vi "Test Graph.vi"() -> ()   [LabVIEW 2020]
uses:
  <vilib>/Utility/cursorutil.llb/Set Cursor (Icon Pict).vi
  <vilib>/Utility/miscctls.llb/LVPoint32TypeDef.ctl
panel:
  out "x/y":sgl
  in  "数值 2":dbl
  in  "数值":dbl
  in  "最小精度":enum32{"1min", "10s", "1s", "100ms"}(radio)
  in  "Process":bool
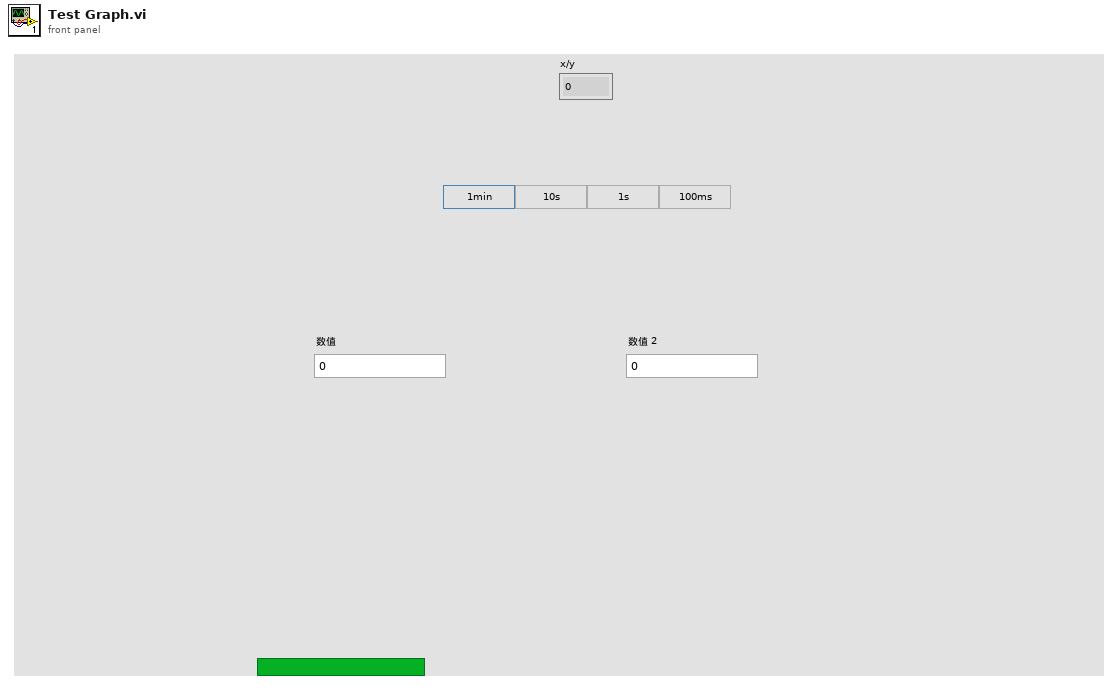
[diagram p1: front panel]
types:
  T1 = typedef "LVPoint32TypeDef.ctl" = cluster{"Horizontal":i32, "Vertical":i32}
  T2 = enum32{"invalid app kind", "Development System", "Run Time System", "Student Edition", "Embedded LabVIEW", "Evaluation", "Custom"}
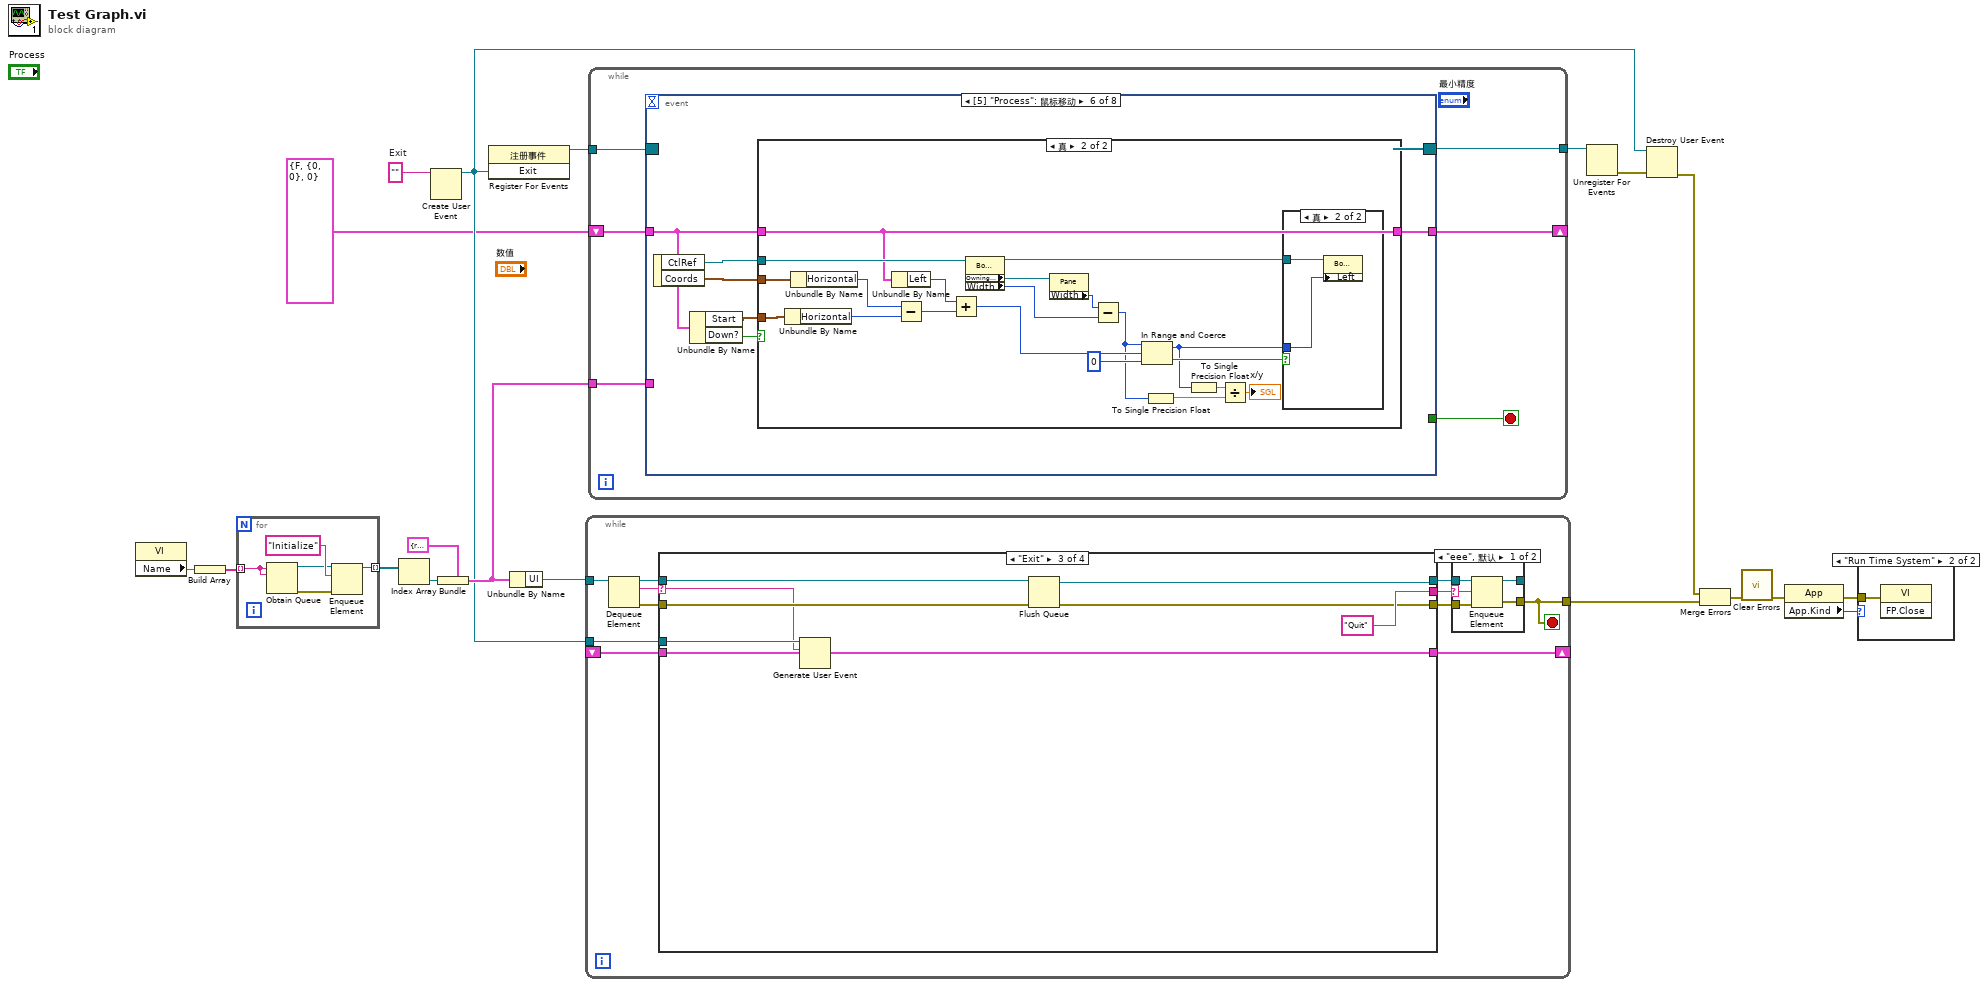
[diagram p0: block diagram]
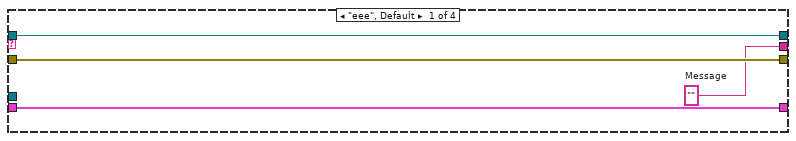
[diagram p4: hidden frame]
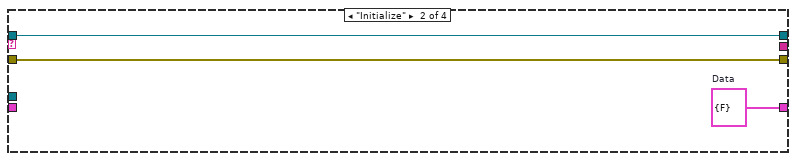
[diagram p5: hidden frame]
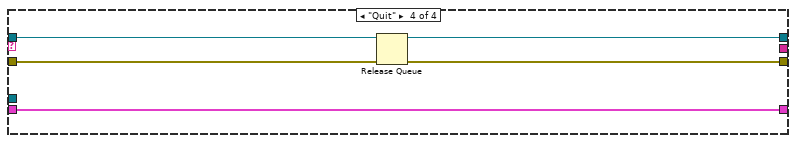
[diagram p6: hidden frame]
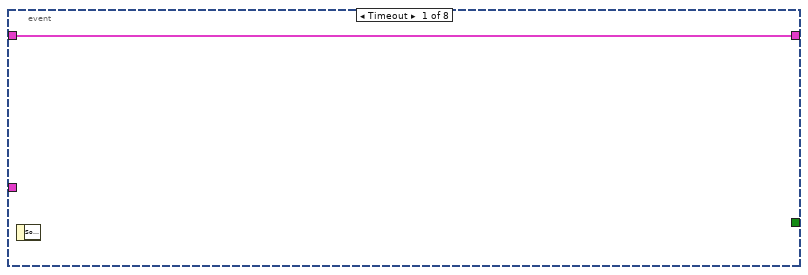
[diagram p7: hidden frame]
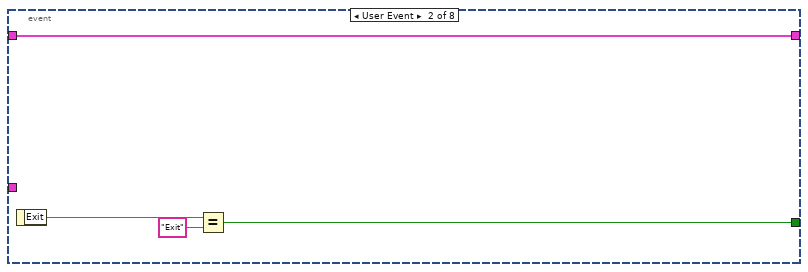
[diagram p8: hidden frame]
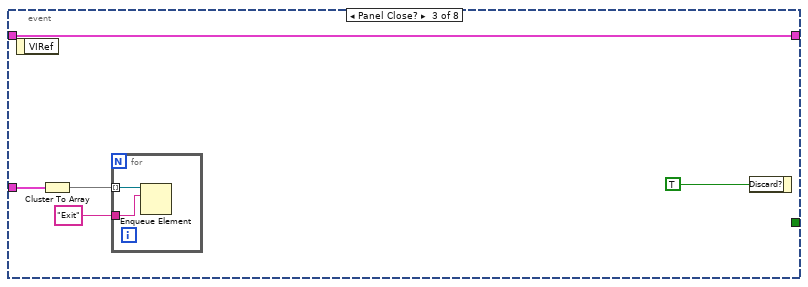
[diagram p9: hidden frame]
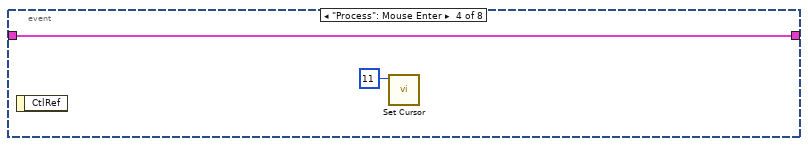
[diagram p10: hidden frame]
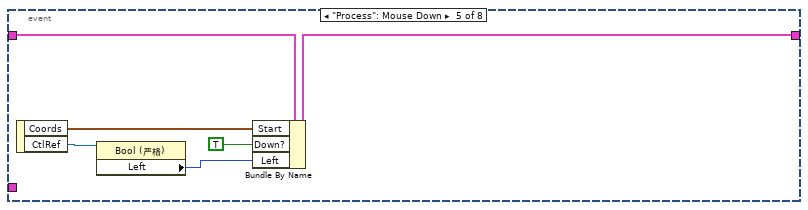
[diagram p11: hidden frame]
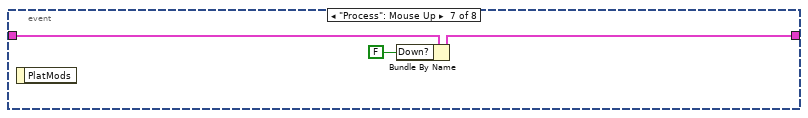
[diagram p14: hidden frame]
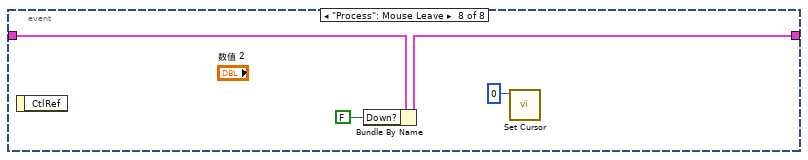
[diagram p15: hidden frame]
diagram:
  w4 = ""  # Exit
  n1 = property class="VI"() -> ("Name"=w14:string)  [unwired: 2 in, 2 out]
  n2 = Build Array(w14) -> (w15:string[])
  n3 = for {
    tunnel: w15 -> [w20] mode=indexing
    tunnel: [w21] -> w9 mode=indexing
    n4 = Obtain Queue(name (unnamed)=w20, element data type=w20) -> (queue out=w23:refnum<queue>, error out=w22:errorcluster)  [unwired: 3 in, 1 out]
    n5 = Enqueue Element(queue=w23, element="Initialize" ("元素"), error in (no error)=w22) -> (queue out=w21:refnum<queue>)  [unwired: 1 in, 2 out]
  }
  n6 = Index Array(array=w9) -> (element=w12:refnum<queue>)  [unwired: 1 in]
  n7 = Create User Event(user event datatype=w4) -> (user event=w8:refnum<user-event>)  [unwired: 1 in, 1 out]
  n8 = Bundle(cluster=cluster{"UI":refnum<queue>} {"UI"=refnum}, "UI"=w12) -> (w13:cluster{"UI":refnum<queue>})
  n9 = register-events(w8) -> (reference out=w5:refnum<event-registration>)  [unwired: 2 in, 1 out]
  n10 = Unbundle By Name(w13) -> ("UI"=w10:refnum<queue>)
  n11 = while {
    tunnel: w10 -> [w35]
    tunnel: [w25] -> w17
    shift-right: [w29] -> _
    shift-left: _ -> [w28]
    tunnel: w8 -> [w27]
    stop <- w25 stop-if-true
    n12 = Dequeue Element(queue=w35) -> (queue out=w34:refnum<queue>, element=w26:string, error out=w31:errorcluster)  [unwired: 2 in, 1 out]
    n13 = case shown="\"Exit\"" w26 {
      selector: w26 -> [_ _ w50 _]
      tunnel: w34 -> [w46 w49 w55 w61]
      tunnel: [w46 w49 w54 w61] -> w33
      tunnel: [w45 w48 w53 w58] -> w32
      tunnel: w31 -> [w45 w48 w52 w60]
      tunnel: [w44 _ "Quit" ("Message") _] -> w30
      tunnel: [w43 w47 w57 w59] -> w29
      tunnel: w28 -> [w43 _ w57 w59]
      tunnel: w27 -> [_ _ w51 _]
      frame "eee", Default {
        w44 = ""  # Message
      }
      frame "Initialize" {
        w47 = cluster{"Data":bool} {"Data"=FALSE}  # Data
      }
      frame "Exit" {
        n14 = Generate User Event(user event=w51, event data cluster=w50) -> ()  [unwired: 2 in, 2 out]
        n15 = Flush Queue(queue=w55, error in (no error)=w52) -> (queue out=w54:refnum<queue>, error out=w53:errorcluster)  [unwired: 1 out]
      }
      frame "Quit" {
        n16 = Release Queue(queue=w61, error in (no error)=w60) -> (error out=w58:errorcluster)  [unwired: 1 in, 2 out]
      }
    }
    n17 = case shown="\"eee\", 默认" w30 {
      selector: w30 -> [w36 _]
      tunnel: w33 -> [w40 w42]
      tunnel: w32 -> [w39 w41]
      tunnel: [w38 w41] -> w25
      tunnel: [w37 w42] -> _
      frame "eee", Default {
        n18 = Enqueue Element(queue=w40, element=w36, error in (no error)=w39) -> (queue out=w37:refnum<queue>, error out=w38:errorcluster)  [unwired: 1 in, 1 out]
      }
      frame "" {
      }
    }
  }
  n19 = while {
    tunnel: w5 -> [w66]
    tunnel: [w65] -> w7
    tunnel: w13 -> [w64]
    shift-right: [w62] -> _
    shift-left: cluster{"Down?":bool, "Start":T1, "Left":i32} {"Down?"=FALSE, "Start"={"Horizontal"=0, "Vertical"=0}, "Left"=0} -> [w63]
    stop <- w67 stop-if-true
    n20 = event shown="[5] \"Process\": 鼠标移动" {
      selector: w66 -> [_ _ _ _ _ _ _ _]
      dyn-events: [_ _ _ _ _ _ _ _] -> w65
      timeout: _ -> [_ _ _ _ _ _ _ _]
      tunnel: [_ w71 _ _ _ _ _ _] -> w67
      tunnel: w64 -> [_ _ w76 _ _ _ _ _]
      tunnel: w63 -> [w68 w69 w73 w80 w87 w92 w119 w122]
      tunnel: [w68 w69 w73 w80 w86 w91 w118 w121] -> w62
      event Timeout {
        n21 = event-data() -> ()  [unwired: 1 in, 1 out]
      }
      event User Event {
        n22 = event-data() -> ("Exit"=w72:string)  [unwired: 1 in]
        n23 = Equal?(x=w72, y="Exit") -> (x = y?=w71:bool)
      }
      event Panel Close? {
        n24 = event-data() -> ()  [unwired: 1 in, 1 out]
        n25 = Cluster To Array(cluster=w76) -> (array=w75:refnum<queue>[])
        n26 = for {
          tunnel: w75 -> [w79] mode=indexing
          tunnel: "Exit" ("元素") -> [w78]
          n27 = Enqueue Element(queue=w79, element=w78) -> ()  [unwired: 2 in, 3 out]
        }
        n28 = event-data("Discard?"=TRUE ("放弃？")) -> ()  [unwired: 1 in, 1 out]
      }
      event "Process": Mouse Enter {
        n29 = event-data() -> ()  [unwired: 1 in, 1 out]
        n30 = call-poly <vilib>:"Set Cursor.vi"("icon"=u16 11) -> ()  [unwired: 9 in, 2 out]
      }
      event "Process": Mouse Down {
        n31 = event-data() -> ("Coords"=w85:T1, "CtlRef"=w83:refnum<vi>)  [unwired: 1 in]
        n32 = property class="Bool (严格)"(reference=w83) -> ("Left"=w82:i32)  [unwired: 1 in, 2 out]
        n33 = Bundle By Name(cluster=w87, "Start"=w85, "Down?"=TRUE, "Left"=w82) -> (w86:cluster{"Down?":bool, "Start":T1, "Left":i32})
      }
      event "Process": Mouse Move {
        n34 = event-data() -> ("CtlRef"=w88:refnum<vi>, "Coords"=w90:T1)  [unwired: 1 in]
        n35 = Unbundle By Name(w92) -> ("Start"=w89:T1, "Down?"=w93:bool)
        n36 = case shown="真" w93 {
          tunnel: w92 -> [w94 w98]
          tunnel: [w94 w98] -> w91
          tunnel: w90 -> [_ w114]
          tunnel: w89 -> [_ w113]
          tunnel: w88 -> [_ w105]
          frame False {
          }
          frame True {
            n37 = Unbundle By Name(w113) -> ("Horizontal"=w111:i32)
            n38 = Unbundle By Name(w114) -> ("Horizontal"=w112:i32)
            n39 = Unbundle By Name(w98) -> ("Left"=w110:i32)
            n40 = Subtract(x=w112, y=w111) -> (x-y=w109:i32)
            n41 = Add(x=w110, y=w109) -> (x+y=w103:i32)
            n42 = property class="Bool (严格)"(reference=w105) -> (reference out=w102:refnum<vi>, "OwningPane"=w107:refnum<vi>, "Width"=w106:u32)  [unwired: 1 in, 1 out]
            n43 = property class="Pane"(reference=w107) -> ("Width"=w108:u32)  [unwired: 1 in, 2 out]
            n44 = Subtract(x=w108, y=w106) -> (x-y=w99:u32)
            n45 = In Range and Coerce(upper limit=w99, x=w103, lower limit=u32 0 ("下限")) -> (coerced(x)=w100:u32, In Range?=w101:bool)
            n46 = To Single Precision Float(number=w99) -> (single precision float=w96:sgl)
            n47 = To Single Precision Float(number=w100) -> (single precision float=w97:sgl)
            n48 = Divide(x=w97, y=w96) -> (x/y=→"x/y":sgl)
            n49 = case shown="真" w101 {
              tunnel: w102 -> [_ w116]
              tunnel: w100 -> [_ w115]
              frame False {
              }
              frame True {
                n50 = property class="Bool (严格)"(reference=w116, "Left"=w115) -> ()  [unwired: 1 in, 2 out]
              }
            }
          }
        }
      }
      event "Process": Mouse Up {
        n51 = event-data() -> ()  [unwired: 1 in, 1 out]
        n52 = Bundle By Name(cluster=w119, "Down?"=FALSE) -> (w118:cluster{"Down?":bool, "Start":T1, "Left":i32})
      }
      event "Process": Mouse Leave {
        n53 = event-data() -> ()  [unwired: 1 in, 1 out]
        n54 = Bundle By Name(cluster=w122, "Down?"=FALSE) -> (w121:cluster{"Down?":bool, "Start":T1, "Left":i32})
        n55 = call-poly <vilib>:"Set Cursor.vi"("icon"=u16 0) -> ()  [unwired: 9 in, 2 out]
      }
    }
  }
  n56 = Unregister For Events(event registration refnum=w7) -> (error out=w6:errorcluster)  [unwired: 1 in]
  n57 = Destroy User Event(user event=w8, error in=w6) -> (error out=w16:errorcluster)
  n58 = Merge Errors(w16, w17) -> (w18:errorcluster)
  n59 = call <vilib>:"Clear Errors.vi"("error in (no error)"=w18) -> ("error out"=w19:errorcluster)  [unwired: 5 in, 1 out]
  n60 = property class="App"(error in=w19) -> (error out=w2:errorcluster, "App.Kind"=w3:T2)  [unwired: 1 in, 1 out]
  n61 = case shown="\"Run Time System\"" w3 {
    tunnel: w2 -> [_ w124]
    frame "invalid app kind", Default {
    }
    frame "Run Time System" {
      n62 = invoke class="VI" method="FP.Close"(error in=w124) -> ()  [unwired: 2 in, 3 out]
    }
  }
